vi "Task Uninit.vi"(8 "error in (no error)":errorcluster, 11 "ChartGuiTask in":refnum<class "ChartGuiTask.lvclass">) -> (0 "error out":errorcluster, 3 "ChartGuiTask out":refnum<class "ChartGuiTask.lvclass">)   [LabVIEW 2020, in "VolatusDemo.lvlib" / "ChartGuiTask.lvclass"]
uses:
  ChartGuiTask.lvclass
  ChartGuiTask.lvclass/ChartGuiTask.ctl
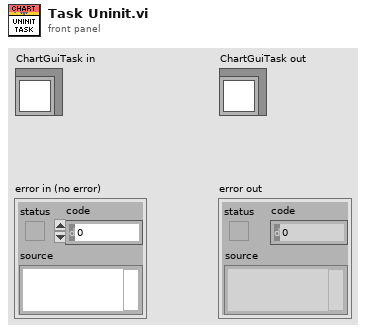
[diagram p1: front panel]
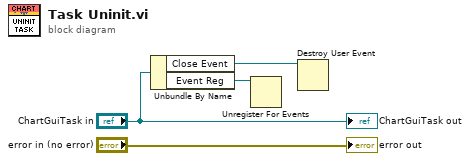
[diagram p0: block diagram]
diagram:
  n1 = Unbundle By Name("ChartGuiTask in") -> ("Close Event"=w1:refnum<user-event>, "Event Reg"=w2:refnum<event-registration>)
  n2 = Unregister For Events(event registration refnum=w2) -> ()  [unwired: 1 in, 1 out]
  n3 = Destroy User Event(user event=w1) -> ()  [unwired: 1 in, 1 out]
  "error out" <- "error in (no error)"
  "ChartGuiTask out" <- "ChartGuiTask in"
